vi "validate.vi"(8 "error in":errorcluster, 11 "Thermo Channel configuration in":refnum<class "Thermo Channel configuration.lvclass">) -> (0 "error out":errorcluster, 3 "Thermo Channel configuration out":refnum<class "Thermo Channel configuration.lvclass">)   [LabVIEW 2025, in "Thermo.lvlib" / "Thermo Channel configuration.lvclass"]
doc: "Provides an interface for performing validation on a given configuration. Any children should define the behavior of this function to ensure that the configuration in memory can be used by the runtime class.Copyright 2017 National Instruments Corporation\n\nLicensed under the Apache License, Version 2.0 (the \"License\"); you may not use this file except in compliance with the License. You may obtain a copy of the License at http://www.apache.org/licenses/LICENSE-2.0\nUnless required by applicable law or agreed to in writing, software distributed under the License is distributed on an \"AS IS\" BASIS, WITHOUT WARRANTIES OR CONDITIONS OF ANY KIND, either express or implied. See the License for the specific language governing permissions and limitations under the License."
uses:
  Thermo Channel configuration.lvclass
  Thermo Channel configuration.lvclass/Thermo Channel configuration.ctl
  Users/Public/Documents/Sandia National Labs/TSS Plugin/CEF.lvlibp
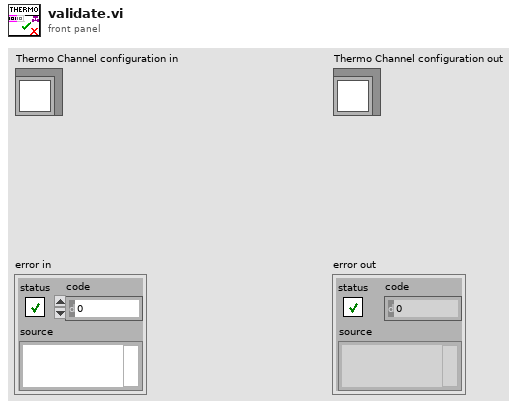
[diagram p1: front panel]
types:
  T1 = cluster{"Address":string, "SW Alias":string, "Enabled":bool, "Type":string, "Description":string}
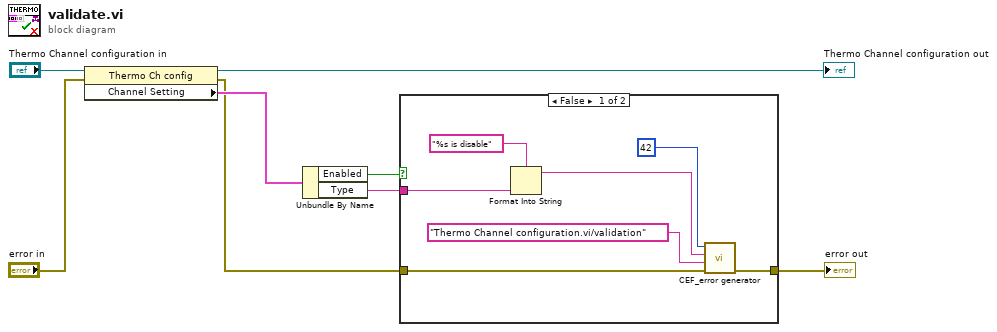
[diagram p0: block diagram]
diagram:
  n1 = property class="Thermo Ch config"(reference="Thermo Channel configuration in", error in="error in") -> (reference out=→"Thermo Channel configuration out":refnum<class "Thermo Channel configuration.lvclass">, error out=w1:errorcluster, "Channel Setting"=w8:T1)
  n2 = Unbundle By Name(w8) -> ("Enabled"=w6:bool, "Type"=w7:string)
  n3 = case shown="False" w6 {
    tunnel: w1 -> [w15 w16]
    tunnel: [w14 w16] -> w4
    tunnel: w7 -> [w11 _]
    frame False {
      n4 = Format Into String(format string="%s is disable" ("append error message"), w11) -> (resulting string=w10:string)  [unwired: 2 in, 1 out]
      n5 = call "CEF_error generator.vi"("error in"=w15, "source"="Thermo Channel configuration.vi/validation", "append error message"=w10, "error code (0)"=42) -> ("error out"=w14:errorcluster)  [unwired: 5 in]
    }
    frame True {
    }
  }
  "error out" <- w4
